vi "Generate PPS at sec boundary and Wait.vi"() -> ()   [LabVIEW 2016]
doc: "This example shows how to configure your Timing and Synchronization board to generate a 1Hz clock pulse train. This clock could be routed to virtual instruments that use a shared trigger bus such as RTSI or traditional instruments via the SMB connector to synchronize a system. The clock pulse generation begins when the current time reaches the specified clock start time. \n\nTo synchronize multiple clocks across 1588, refer to the Generate Sync Clock-Master and Generate Sync Clock-Slave advanced example VIs."
uses:
  <instrlib>/niSync/niSync.llb/niSync Initialize (IVI).vi
  <instrlib>/niSync/niSync.llb/niSync Create Clock (Frequency).vi
panel:
  in  "Output Terminal":tag="PFI0"
  in  "Resource Name":refnum<k15>="PXI1Slot2"
  out "Current Time":timestamp format="%<%I:%M:%S%9u %p\n%x>T"
  in  "stop":bool
  out "Clock Start Time":timestamp format="%<%I:%M:%S%9u %p\n%x>T"
  in  "Start Time Delay (Seconds)":dbl=2.0
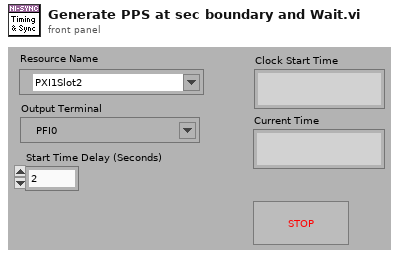
[diagram p1: front panel]
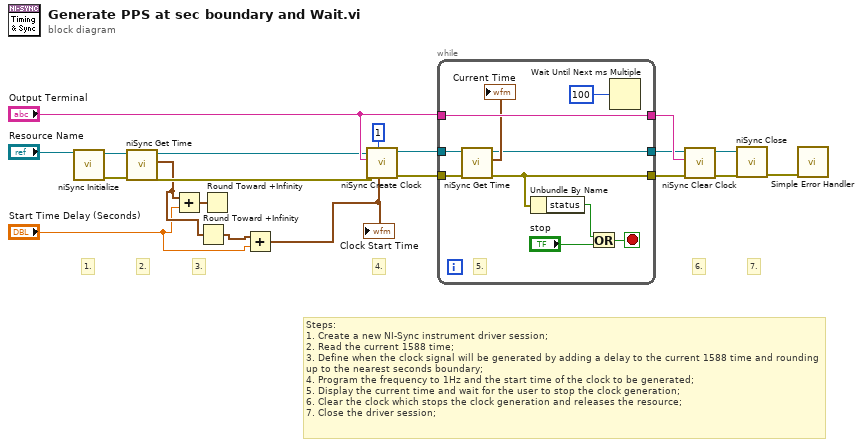
[diagram p0: block diagram]
diagram:
  # "3."
  # "4."
  # "7."
  # "6."
  # "2."
  # "1."
  # "Steps:\n1. Create a new NI-Sync instrument driver session;\n2. Read the current 1588 time;\n3. Define when the clock signal will be generated by adding a delay to the current 1588 time and rounding up to the nearest seconds boundary;\n4. Program the frequency to 1Hz and the start time of the clock to be generated; \n5. Display the current time and wait for the user to stop the clock generation;\n6. Clear the clock which stops the clock generation and releases the resource;\n7. Close the driver session;"
  n1 = call-poly <instrlib>:"niSync Initialize.vi"("resource name"="Resource Name") -> ("error out"=w16:errorcluster, "instrument handle out"=w11:refnum<k15>)  [unwired: 9 in]
  n2 = call <instrlib>:"niSync Get Time.vi"("error in (no error)"=w16, "instrument handle"=w11) -> ("error out"=w7:errorcluster, "time"=w4:timestamp, "instrument handle out"=w8:refnum<k15>)  [unwired: 5 in]
  n3 = Add(x=w4, y="Start Time Delay (Seconds)") -> (x+y=w5:timestamp)
  n4 = Round Toward +Infinity(x=w4) -> (ceil(x): smallest int >= x=w3:timestamp)
  n5 = Round Toward +Infinity(x=w5) -> ()  [unwired: 1 out]
  n6 = Add(x=w3, y="Start Time Delay (Seconds)") -> (x+y=w1:timestamp)
  "Clock Start Time" <- w1
  n7 = call-poly <instrlib>:"niSync Create Clock.vi"("start time"=w1, "frequency"=u32 1 ("Desired Clock Frequency (Hz)"), "error in (no error)"=w7, "terminal"="Output Terminal", "instrument handle"=w8) -> ("error out"=w18:errorcluster, "instrument handle out"=w19:refnum<k15>)  [unwired: 3 in, 2 out]
  n8 = while {
    tunnel: w19 -> [w25]
    tunnel: w18 -> [w26]
    tunnel: [w27] -> w17
    tunnel: "Output Terminal" -> [w27]
    tunnel: [w23] -> w15
    tunnel: [w22] -> w14
    stop <- w29 stop-if-true
    # "5."
    n9 = call <instrlib>:"niSync Get Time.vi"("error in (no error)"=w26, "instrument handle"=w25) -> ("error out"=w22:errorcluster, "time"=→"Current Time":timestamp, "instrument handle out"=w23:refnum<k15>)  [unwired: 5 in]
    n10 = Unbundle By Name(w22) -> ("status"=w21:bool)
    n11 = Or(x=w21, y="stop") -> (x .or. y?=w29:bool)
    n12 = Wait Until Next ms Multiple(millisecond multiple=u32 100) -> ()  [unwired: 1 out]
  }
  n13 = call <instrlib>:"niSync Clear Clock.vi"("error in (no error)"=w14, "terminal"=w17, "instrument handle"=w15) -> ("error out"=w13:errorcluster, "instrument handle out"=w12:refnum<k15>)  [unwired: 6 in]
  n14 = call <instrlib>:"niSync Close.vi"("error in (no error)"=w13, "instrument handle"=w12) -> ("error out"=w20:errorcluster)  [unwired: 9 in]
  n15 = call <vilib>:"Simple Error Handler.vi"("error in (no error)"=w20) -> ()  [unwired: 4 in, 5 out]
